vi "DBL to string.vi"(11 "Numeric":dbl) -> (3 "F-format string":string)   [LabVIEW 2017]
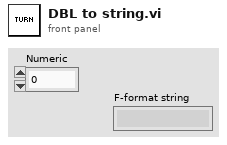
[diagram p1: front panel]
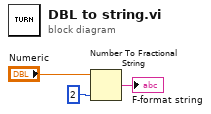
[diagram p0: block diagram]
diagram:
  n1 = Number To Fractional String(number="Numeric", precision (6)=i16 2) -> (F-format string=→"F-format string":string)  [unwired: 2 in]
